vi "Set Voltage.vi"(0 "reference in":refnum<class "Simulated-PowerModule.lvclass">, 5 "voltage (V)":dbl, 11 "Error In":errorcluster) -> (4 "reference out":refnum<class "Simulated-PowerModule.lvclass">, 15 "Error Out":errorcluster)   [LabVIEW 2023, in "Simulated-PowerModule.lvlib" / "Simulated-PowerModule.lvclass"]
uses:
  Simulated-PowerModule.lvclass
  Simulated-PowerModule.lvclass/Simulated-PowerModule.ctl
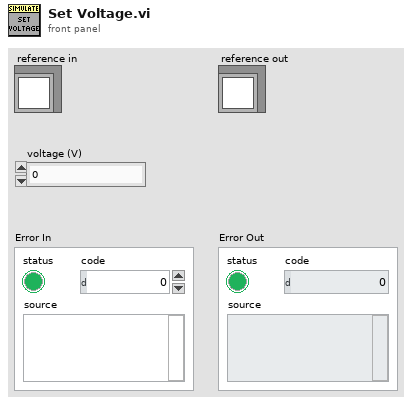
[diagram p1: front panel]
types:
  T1 = typedef "Simulated-PowerModule.lvlib/Simulated-PowerModule.lvclass/ObjectAttributes.ctl" = cluster{"JSON Config Path":path, "Configuration":T2, "connected":bool, "reserved":bool, "energized":bool, "output enabled":bool, "Mode":T3, "Range":T4, "Slew Rates":T5, "Setpoints":cluster{"voltage":dbl, "current":dbl, "resistance":dbl}, "Measurements":cluster{"voltage":dbl, "current":dbl, "resistance":dbl}, "Limits":T6, "active faults":string[], "fault":bool}
  T2 = typedef "Simulated-PowerModule.lvlib/Simulated-PowerModule.lvclass/Configuration.ctl" = cluster{"IP Address":string}
  T3 = typedef "Simulated-PowerModule.lvlib/Simulated-PowerModule.lvclass/Mode.ctl" = u16
  T4 = typedef "PowerModuleInterface.lvlibp/PowerModuleInterface.lvclass/Range.ctl" = cluster{"Current Max (A)":dbl, "Current Min (A)":dbl, "Voltage Max (V)":dbl, "Voltage Min (V)":dbl}
  T5 = typedef "PowerModuleInterface.lvlibp/PowerModuleInterface.lvclass/Slew Rates.ctl" = cluster{"Current Decrease (A/sec)":dbl, "Current Increase (A/sec)":dbl, "Voltage Decrease (V/sec)":dbl, "Voltage Increase (V/sec)":dbl, "Resistance Decrease (Ohm/sec)":dbl, "Resistance Increase (Ohm/sec)":dbl}
  T6 = typedef "PowerModuleInterface.lvlibp/PowerModuleInterface.lvclass/Limits.ctl" = cluster{"Current Max (A)":dbl, "Current Min (A)":dbl, "Voltage Max (V)":dbl, "Voltage Min (V)":dbl, "Power Max (W)":dbl, "Power Min (W)":dbl}
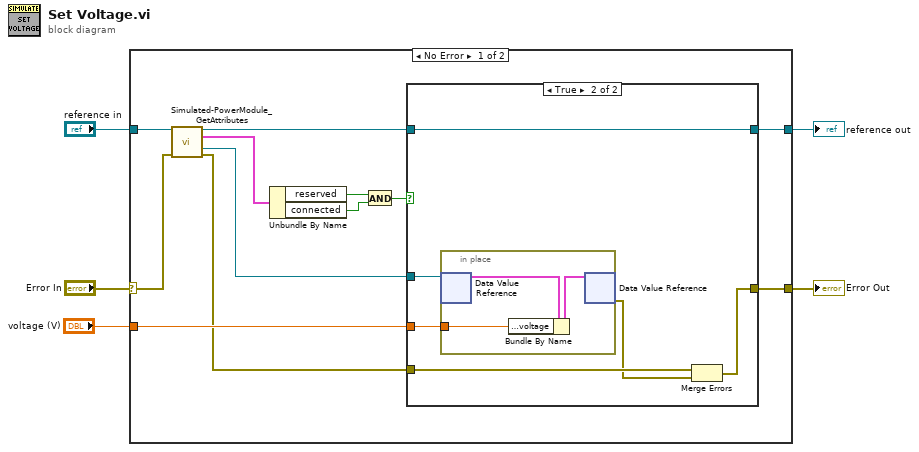
[diagram p0: block diagram]
diagram:
  n1 = case shown="No Error" "Error In" {
    selector: "Error In" -> [w16 w29]
    tunnel: "reference in" -> [w17 w30]
    tunnel: [w13 w30] -> w2
    tunnel: [w12 w29] -> w3
    tunnel: "voltage (V)" -> [w11 _]
    frame No Error {
      n2 = call "Simulated-PowerModule_GetAttributes.vi"("reference in"=w17, "Error In"=w16) -> ("reference out"=w14:refnum<class "Simulated-PowerModule.lvclass">, "Data"=w10:T1, "DataRef"=w15:refnum<data-value>, "Error Out"=w9:errorcluster)  [unwired: 10 in]
      n3 = Unbundle By Name(w10) -> ("reserved"=w8:bool, "connected"=w7:bool)
      n4 = And(x=w8, y=w7) -> (x .and. y?=w6:bool)
      n5 = case shown="True" w6 {
        tunnel: w15 -> [_ w25]
        tunnel: w14 -> [w19 w24]
        tunnel: [w19 w24] -> w13
        tunnel: [w18 w20] -> w12
        tunnel: w11 -> [_ w23]
        tunnel: w9 -> [w18 w22]
        frame False {
        }
        frame True {
          n6 = in-place {
            in-place-border: w23 -> [w26]
            n7 = in-place-dvr #1(w25) -> (w28:T1)  [unwired: 1 out]
            n8 = Bundle By Name(cluster=w28, "Setpoints.voltage"=w26) -> (w27:T1)
            n9 = in-place-dvr #1(w27) -> (w21:errorcluster)  [unwired: 1 out]
          }
          n10 = Merge Errors(w22, w21) -> (w20:errorcluster)
        }
      }
    }
    frame Error {
    }
  }
  "Error Out" <- w3
  "reference out" <- w2
